vi "helper-serial-log-to-string-2.vi"(10 "filter":T7, 11 "Array in":T1[](array[typedef]) {"IOnode"."calibration"."Y" format="%#.3f"; "IOnode"."calibration"."X" format="%#.3f"; "IOnode"."ADDR" format="%04d"}) -> (3 "Array out":T7[](array[typedef]))   [LabVIEW 2024]
uses:
  controls/eng-serial-log.ctl
  controls/cluster-com-log.ctl
  controls/IONode.ctl
  controls/type.address.ctl
  controls/enum.io.type.ctl
  controls/enum.io.mode.ctl
  controls/typeXyPoint.ctl
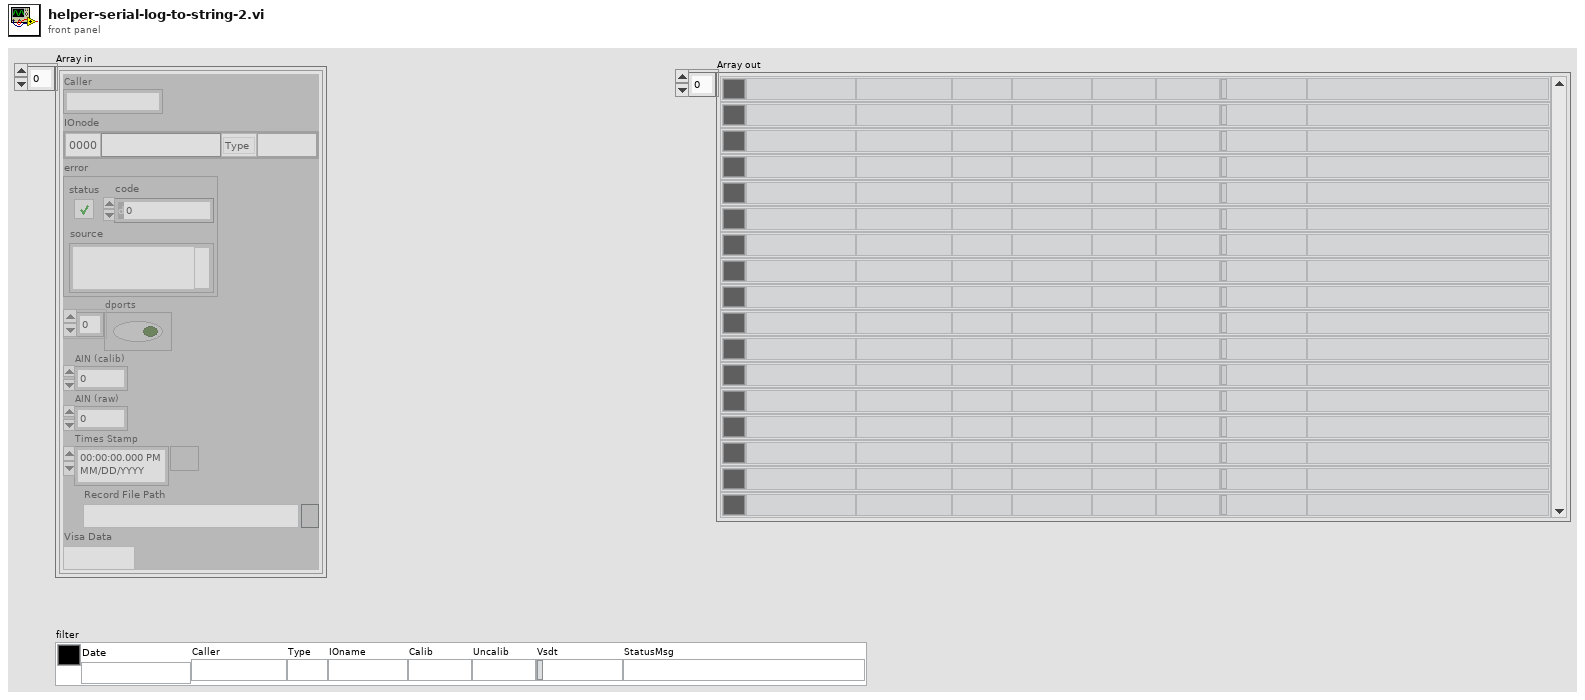
[diagram p1: front panel]
types:
  T1 = typedef "cluster-com-log.ctl" = cluster{"Caller":string, "IOnode":T2, "error":errorcluster, "dports":bool[], "AIN (calib)":dbl, "AIN (raw)":u16, "Times Stamp":timestamp, "Record File Path":path, "Visa Data":string}
  T2 = typedef "IONode.ctl" = cluster{"ADDR":T3, "Label":string, "Type":T4, "Mode":T5, "Value":string, "Tags":string, "calibration":T6[]}
  T3 = typedef "type.address.ctl" = u16
  T4 = typedef "enum.io.type.ctl" = enum16{"Type", "DI", "DO", "AI", "AO", "VL", "BUF"}
  T5 = typedef "enum.io.mode.ctl" = enum16{"Mode", "RIO", "SIM"}
  T6 = typedef "typeXyPoint.ctl" = cluster{"X":dbl, "Y":dbl}
  T7 = typedef "eng-serial-log.ctl" = cluster{"Status":u32, "Date":string, "Caller":string, "Type":string, "IOname":string, "Calib":string, "Uncalib":string, "Vsdt":string, "StatusMsg":string}
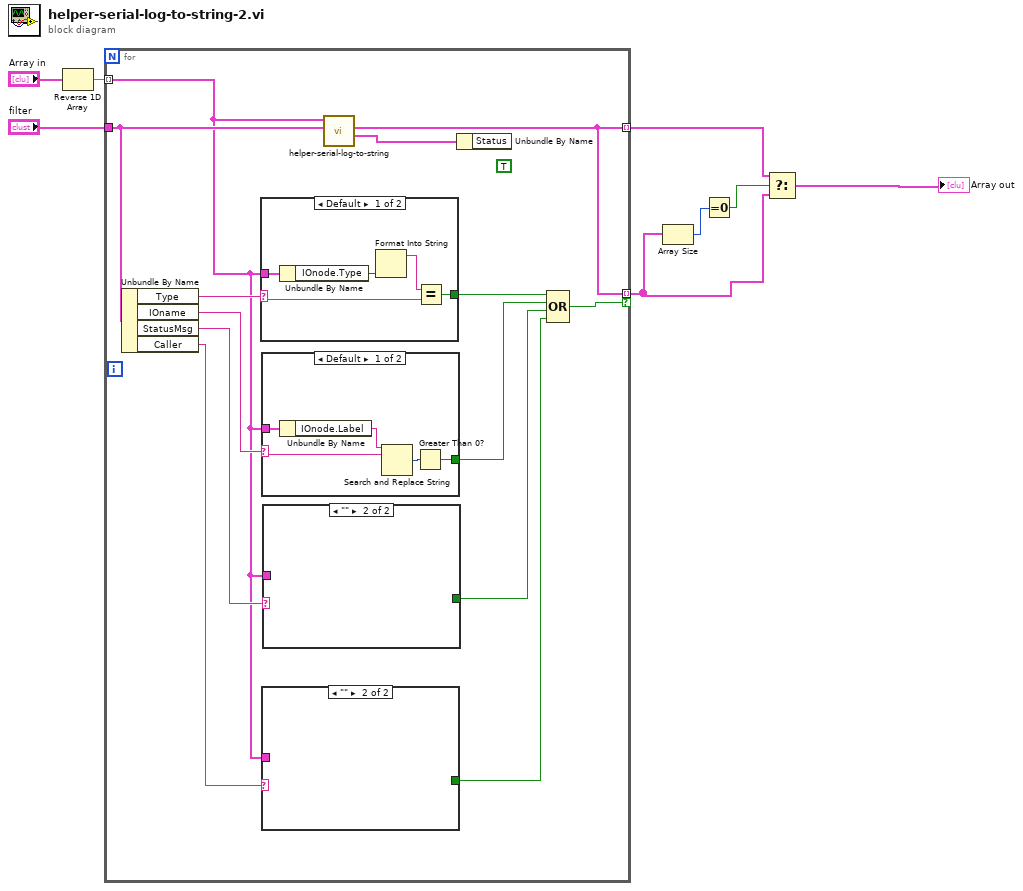
[diagram p0: block diagram]
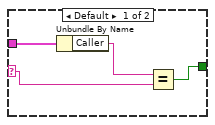
[diagram p2: hidden frame]
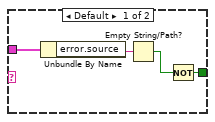
[diagram p3: hidden frame]
diagram:
  n1 = Reverse 1D Array(array="Array in") -> (reversed array=w7:T1[])
  n2 = for {
    tunnel: w7 -> [w11] mode=indexing
    tunnel: [w12] -> w2 mode=indexing if=w13
    tunnel: "filter" -> [w20]
    tunnel: [w12] -> w3 mode=indexing
    (unwired) TRUE
    n3 = Unbundle By Name(w20) -> ("Type"=w19:string, "IOname"=w17:string, "StatusMsg"=w15:string, "Caller"=w10:string)
    n4 = case shown="Default" w19 {
      selector: w19 -> [w36 _]
      tunnel: w11 -> [w39 _]
      tunnel: [w35 _] -> w18
      frame Default {
        n5 = Unbundle By Name(w39) -> ("IOnode.Type"=w38:T4)
        n6 = Format Into String(w38) -> (resulting string=w37:string)  [unwired: 3 in, 1 out]
        n7 = Equal?(x=w37, y=w36) -> (x = y?=w35:bool)
      }
      frame "" {
      }
    }
    n8 = case shown="Default" w17 {
      selector: w17 -> [w31 _]
      tunnel: w11 -> [w34 _]
      tunnel: [w33 _] -> w16
      frame Default {
        n9 = Unbundle By Name(w34) -> ("IOnode.Label"=w32:string)
        n10 = Search and Replace String(input string=w32, search string=w31) -> (number of replacements=w30:i32)  [unwired: 6 in, 3 out]
        n11 = Greater Than 0?(x=w30) -> (x > 0?=w33:bool)
      }
      frame "" {
      }
    }
    n12 = case shown="\"\"" w10 {
      selector: w10 -> [w23 _]
      tunnel: [w22 _] -> w9
      tunnel: w11 -> [w25 _]
      frame Default {
        n13 = Unbundle By Name(w25) -> ("Caller"=w24:string)
        n14 = Equal?(x=w24, y=w23) -> (x = y?=w22:bool)
      }
      frame "" {
      }
    }
    n15 = case shown="\"\"" w15 {
      tunnel: [w26 _] -> w14
      tunnel: w11 -> [w29 _]
      frame Default {
        n16 = Unbundle By Name(w29) -> ("error.source"=w28:string)
        n17 = Empty String/Path?(string/path=w28) -> (empty?=w27:bool)
        n18 = Not(x=w27) -> (.not. x?=w26:bool)
      }
      frame "" {
      }
    }
    n19 = call "helper-serial-log-to-string.vi"("filter"=w20, "input cluster"=w11) -> ("output cluster"=w21:cluster{"Status":bool}, "Snapshot"=w12:T7)  [unwired: 7 in, 1 out]
    n20 = Unbundle By Name(w21) -> ()  [unwired: 1 out]
    n21 = Compound Arithmetic op=OR(w18, w16, w14, w9) -> (w13:bool)
  }
  n22 = Array Size(array=w2) -> (size(s)=w4:i32)
  n23 = Equal To 0?(x=w4) -> (x = 0?=w5:bool)
  n24 = Select(t=w3, s=w5, f=w2) -> (s? t:f=→"Array out":T7[])
